vi "Client Cancel Call.vi"(8 "error in":errorcluster, 11 "Call ID in":T1) -> (0 "error out":errorcluster, 1 "errorDetails":T2, 3 "Call ID out":T1)   [LabVIEW 2019, in "grpc-lvsupport.lvlib"]
uses:
  grpc-lvsupport.lvlib
  grpcId.ctl
  Any.ctl
  <vilib>/Utility/error.llb/Error Cluster From Error Code.vi
  <resource>/labview_grpc_server.dll
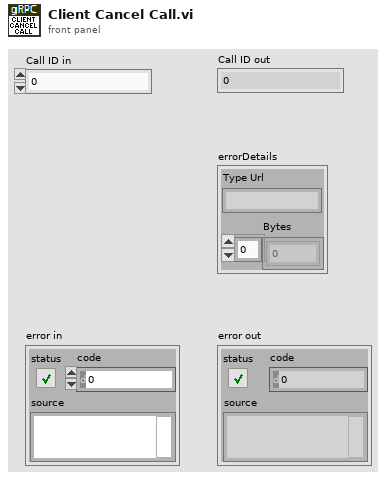
[diagram p1: front panel]
types:
  T1 = typedef "grpc-lvsupport.lvlib/grpcId.ctl" = u64
  T2 = typedef "grpc-lvsupport.lvlib/Any.ctl" = cluster{"Type Url":string, "Bytes":u8[]}
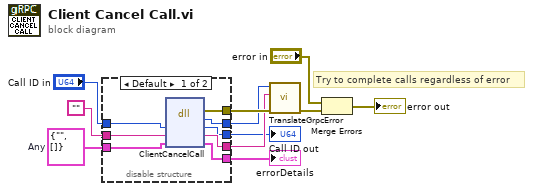
[diagram p0: block diagram]
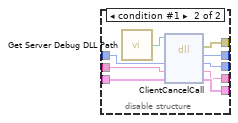
[diagram p2: hidden frame]
diagram:
  w9 = T2 {"Type Url"="", "Bytes"=[]}  # Any
  # "Try to complete calls regardless of error"
  n1 = disable-structure shown="Default" {
    disable-tunnel: [w19 w28] -> w11
    disable-tunnel: "Call ID in" -> [w18 w27]
    disable-tunnel: w9 -> [w17 w26]
    disable-tunnel: [w16 w25] -> w8
    disable-tunnel: [w15 w24] -> w7
    disable-tunnel: [w14 w23] -> w6
    disable-tunnel: [w13 w22] -> w2
    disable-tunnel: "" -> [w12 w21]
    frame condition #0 (active) {
      n2 = dll-call lib="C:/Program Files (x86)/National Instruments/LabVIEW 2024/resource/labview_grpc_server.*" fn="ClientCancelCall"("ClientId"=w18, "errorMessage"=w12, "errorDetails"=w17) -> (error out=w19:errorcluster, "return type"=w14:i32, "ClientId"=w13:u64, "errorMessage"=w15:string, "errorDetails"=w16:T2)  [unwired: 3 in, 1 out]
    }
    frame condition #1 {
      n3 = call "Get Server Debug DLL Path.vi"() -> ("DLL Path"=w20:path)
      n4 = dll-call lib="?" fn="ClientCancelCall"(path in=w20, "ClientId"=w27, "errorMessage"=w21, "errorDetails"=w26) -> (error out=w28:errorcluster, "return type"=w23:i32, "ClientId"=w22:u64, "errorMessage"=w24:string, "errorDetails"=w25:T2)  [unwired: 2 in, 1 out]
    }
  }
  "errorDetails" <- w8
  "Call ID out" <- w2
  n5 = call "TranslateGrpcError.vi"("error in"=w11, "Error Message"=w7, "Error Code"=w6) -> ("error out"=w5:errorcluster)  [unwired: 8 in]
  n6 = Merge Errors("error in", w5) -> (→"error out":errorcluster)
